vi "ROI parser_example.vi"(5 "Circle spot":dbl, 6 "Circle?":bool, 7 "ROI (8 bit image)":u8[][](array[numeric]), 8 "Ablation spot width":i32, 9 "Sampling\nPrecision":dbl, 10 "Ablation spot heigth":i32, 11 "Height  step \ndivider":i32=2) -> (3 "Parsed array":bool[][](array[boolean]))   [LabVIEW 2016]
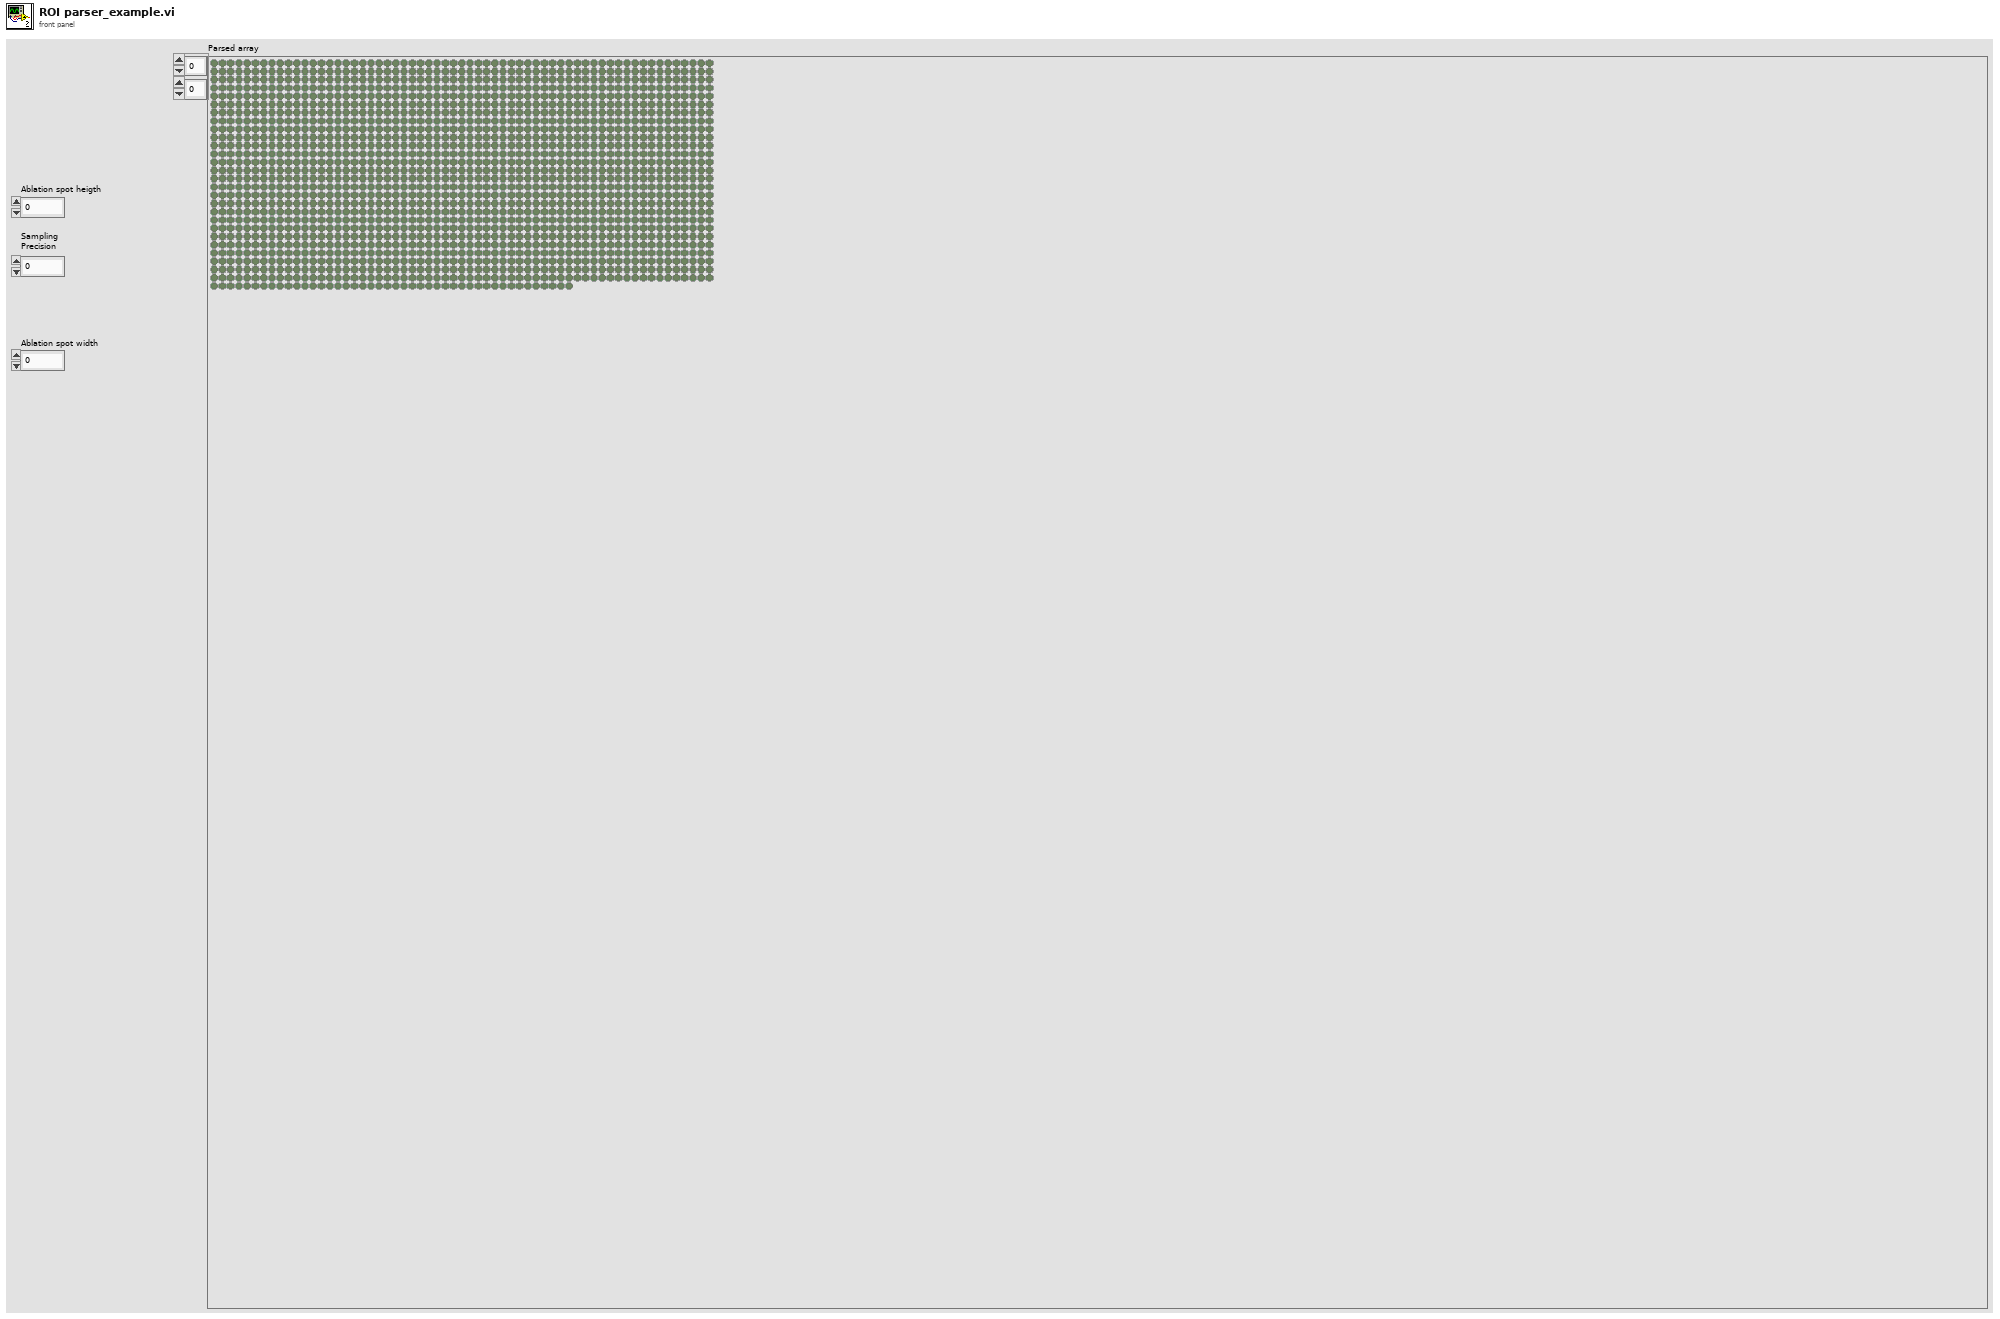
[diagram p1: front panel]
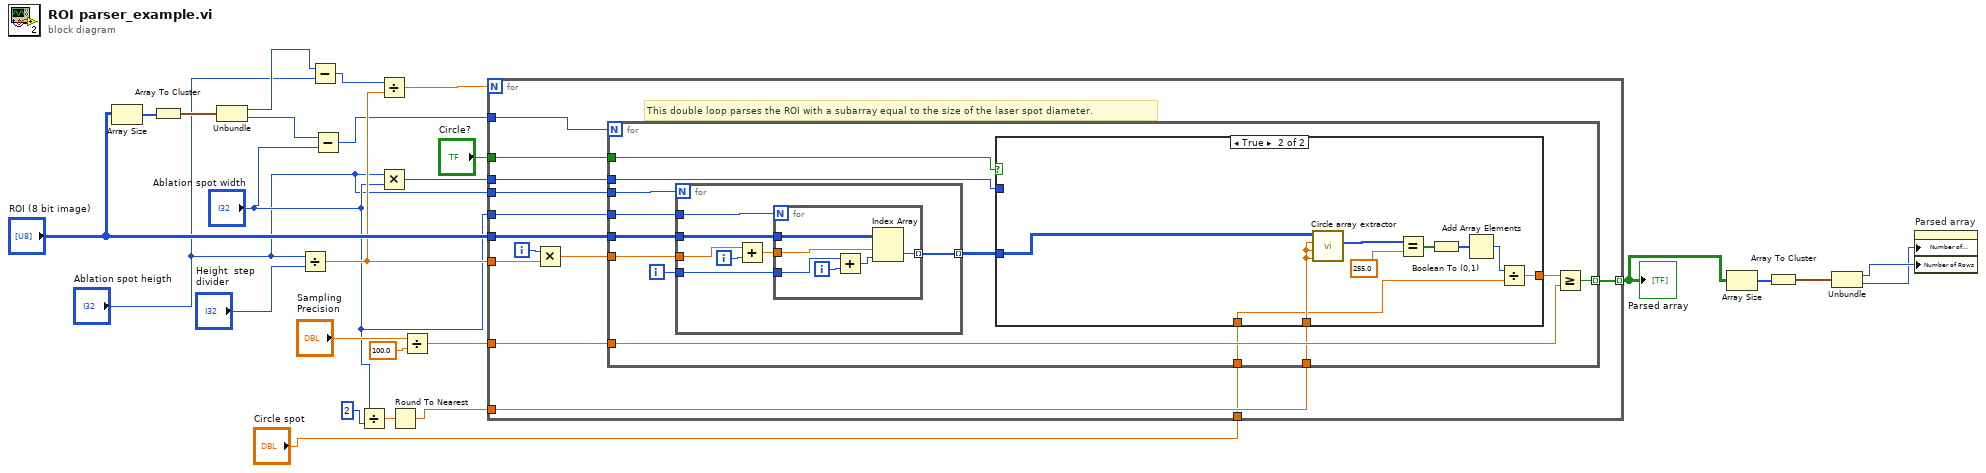
[diagram p0: block diagram]
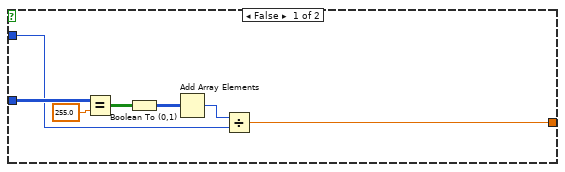
[diagram p2: hidden frame]
diagram:
  n1 = Array Size(array="ROI (8 bit image)") -> (size(s)=w25:i32[])
  n2 = Array To Cluster(array=w25) -> (cluster=w26:cluster{"[0]":i32, "[1]":i32})
  n3 = Unbundle(w26) -> ("[0]"=w3:i32, "[1]"=w10:i32)
  n4 = Divide(x="Ablation spot heigth", y="Height  step \ndivider") -> (x/y=w21:dbl)
  n5 = Subtract(x=w3, y="Ablation spot heigth") -> (x-y=w1:i32)
  n6 = Subtract(x=w10, y="Ablation spot width") -> (x-y=w9:i32)
  n7 = Divide(x="Ablation spot width", y=2 ("x")) -> (x/y=w15:dbl)
  n8 = Divide(x=w1, y=w21) -> (x/y=w22:dbl)
  n9 = Multiply(x="Ablation spot heigth", y="Ablation spot width") -> (x*y=w20:i32)
  n10 = Round To Nearest(number=w15) -> (nearest integer value=w13:dbl)
  n11 = Divide(x="Sampling\nPrecision", y=100.0) -> (x/y=w19:dbl)
  n12 = for {
    N: w22 -> [_]
    tunnel: "ROI (8 bit image)" -> [w39]
    tunnel: "Ablation spot heigth" -> [w38]
    tunnel: [w37] -> w6 mode=indexing
    tunnel: w21 -> [w34]
    tunnel: "Ablation spot width" -> [w33]
    tunnel: w20 -> [w32]
    tunnel: w19 -> [w31]
    tunnel: w9 -> [w30]
    tunnel: "Circle?" -> [w29]
    tunnel: w13 -> [w28]
    tunnel: "Circle spot" -> [w27]
    i -> [w36]
    # "This double loop parses the ROI with a subarray equal to the size of the laser spot diameter."
    n13 = Multiply(x=w36, y=w34) -> (x*y=w35:dbl)
    n14 = for {
      N: w30 -> [_]
      tunnel: w38 -> [w50]
      tunnel: w35 -> [w52]
      tunnel: w39 -> [w51]
      tunnel: [w49] -> w37 mode=indexing
      tunnel: w33 -> [w45]
      tunnel: w32 -> [w44]
      tunnel: w31 -> [w43]
      tunnel: w29 -> [w42]
      tunnel: w28 -> [w41]
      tunnel: w27 -> [w40]
      i -> [w47]
      n15 = for {
        N: w50 -> [_]
        tunnel: w51 -> [w75]
        tunnel: [w74] -> w46 mode=indexing
        tunnel: w45 -> [w73]
        tunnel: w52 -> [w72]
        tunnel: w47 -> [w69]
        i -> [w71]
        n16 = Add(x=w72, y=w71) -> (x+y=w70:dbl)
        n17 = for {
          N: w73 -> [_]
          tunnel: w75 -> [w81]
          tunnel: [w80] -> w74 mode=indexing
          tunnel: w70 -> [w79]
          tunnel: w69 -> [w77]
          i -> [w78]
          n18 = Add(x=w77, y=w78) -> (x+y=w76:i32)
          n19 = Index Array(array=w81, index (row)=w79, index (col)=w76) -> (element=w80:u8)
        }
      }
      n20 = case shown="True" w42 {
        tunnel: [w56 w62] -> w48
        tunnel: w46 -> [w55 w68]
        tunnel: w44 -> [w54 _]
        tunnel: w41 -> [_ w61]
        tunnel: w40 -> [_ w60]
        frame False {
          n21 = Equal?(x=w55, y=255.0) -> (x = y?=w58:bool[][])
          n22 = Boolean To (0,1)(Boolean=w58) -> (0, 1=w57:i16[][])
          n23 = Add Array Elements(numeric array=w57) -> (sum=w53:i16)
          n24 = Divide(x=w53, y=w54) -> (x/y=w56:dbl)
        }
        frame True {
          n25 = call "Circle array extractor.vi"("Center Y"=w61, "Radius"=w61, "Center X"=w61, "initialized array"=w68) -> ("Array 2"=w64:i32[])  [unwired: 6 in]
          n26 = Equal?(x=w64, y=255.0) -> (x = y?=w66:bool[])
          n27 = Boolean To (0,1)(Boolean=w66) -> (0, 1=w65:i16[])
          n28 = Add Array Elements(numeric array=w65) -> (sum=w63:i16)
          n29 = Divide(x=w63, y=w60) -> (x/y=w62:dbl)
        }
      }
      n30 = Greater Or Equal?(x=w48, y=w43) -> (x >= y?=w49:bool)
    }
  }
  "Parsed array" <- w6
  n31 = Array Size(array=w6) -> (size(s)=w7:i32[])
  n32 = Array To Cluster(array=w7) -> (cluster=w8:cluster{"[0]":i32, "[1]":i32})
  n33 = Unbundle(w8) -> ("[0]"=w5:i32, "[1]"=w4:i32)
  n34 = property on="Parsed array" class="Arr (strict)"("Number of Columns"=w4, "Number of Rows"=w5) -> ()  [unwired: 2 in, 2 out]
